vi "G4InterfaceTemplate_6x8x6_Method.vi"(0 "Interface In":refnum<class "G4InterfaceTemplate_6x8x6.lvclass">, 5 "error in (no error)":errorcluster) -> (14 "Interface Out":refnum<class "G4InterfaceTemplate_6x8x6.lvclass">, 19 "error out":errorcluster)   [LabVIEW 2020]
uses:
  <resource>/Framework/Providers/Open_GDS/ClassProviders/Provider_EndevoGOOP400/Templates/G4InterfaceTemplate_6x8x6/G4InterfaceTemplate_6x8x6.lvclass
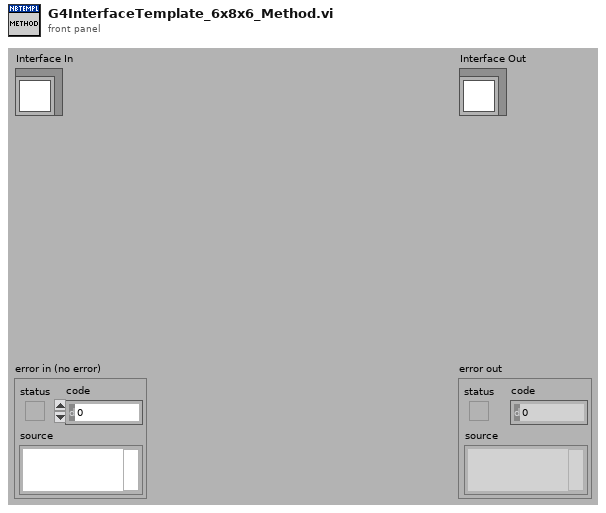
[diagram p1: front panel]
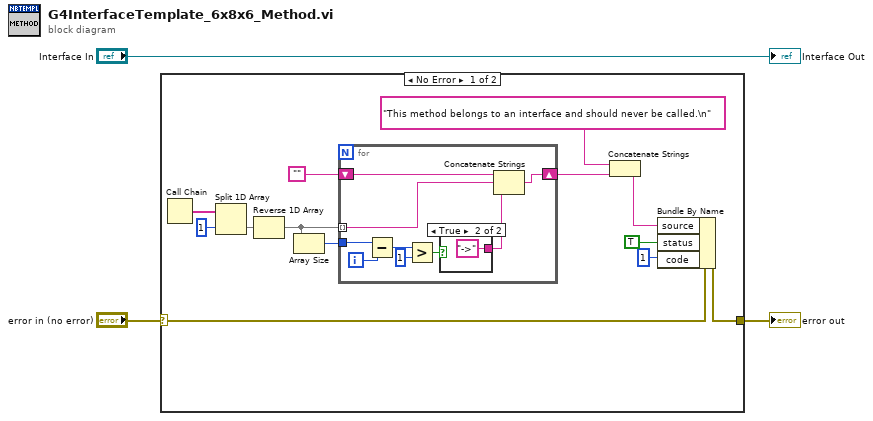
[diagram p0: block diagram]
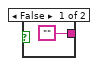
[diagram p2: hidden frame]
diagram:
  n1 = case shown="No Error" "error in (no error)" {
    selector: "error in (no error)" -> [w8 w28]
    tunnel: [w7 w28] -> w1
    frame No Error {
      n2 = Call Chain() -> (call chain=w16:string[])
      n3 = Split 1D Array(array=w16, index=1) -> (second subarray=w14:string[])  [unwired: 1 out]
      n4 = Reverse 1D Array(array=w14) -> (reversed array=w11:string[])
      n5 = Array Size(array=w11) -> (size(s)=w13:i32)
      n6 = for {
        shift-right: [w17] -> w9
        shift-left: "" -> [w20]
        tunnel: w11 -> [w18] mode=indexing
        tunnel: w13 -> [w25]
        i -> [w24]
        n7 = Subtract(x=w25, y=w24) -> (x-y=w23:i32)
        n8 = Greater?(x=w23, y=1) -> (0:w21:bool)
        n9 = case shown="True" w21 {
          tunnel: ["" "->"] -> w19
          frame False {
          }
          frame True {
          }
        }
        n10 = Concatenate Strings(w20, w18, w19) -> (w17:string)
      }
      n11 = Concatenate Strings("This method belongs to an interface and should never be called.\n" ("string"), w9) -> (w6:string)
      n12 = Bundle By Name(cluster=w8, "source"=w6, "status"=TRUE, "code"=1) -> (w7:errorcluster)
    }
    frame Error {
    }
  }
  "error out" <- w1
  "Interface Out" <- "Interface In"
